vi "Nfocus driver V1.2.vi"(5 "error in":errorcluster, 8 "Refs In":T1) -> (0 "error out":errorcluster)   [LabVIEW 2016]
panel:
  out "Running":bool
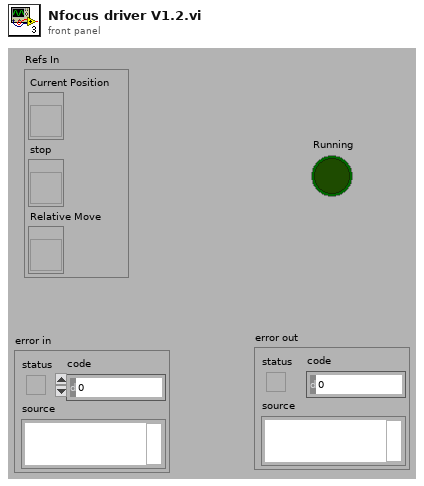
[diagram p1: front panel]
types:
  T1 = cluster{"Current Position":refnum<vi>, "stop":refnum<vi>, "Relative Move":refnum<vi>}
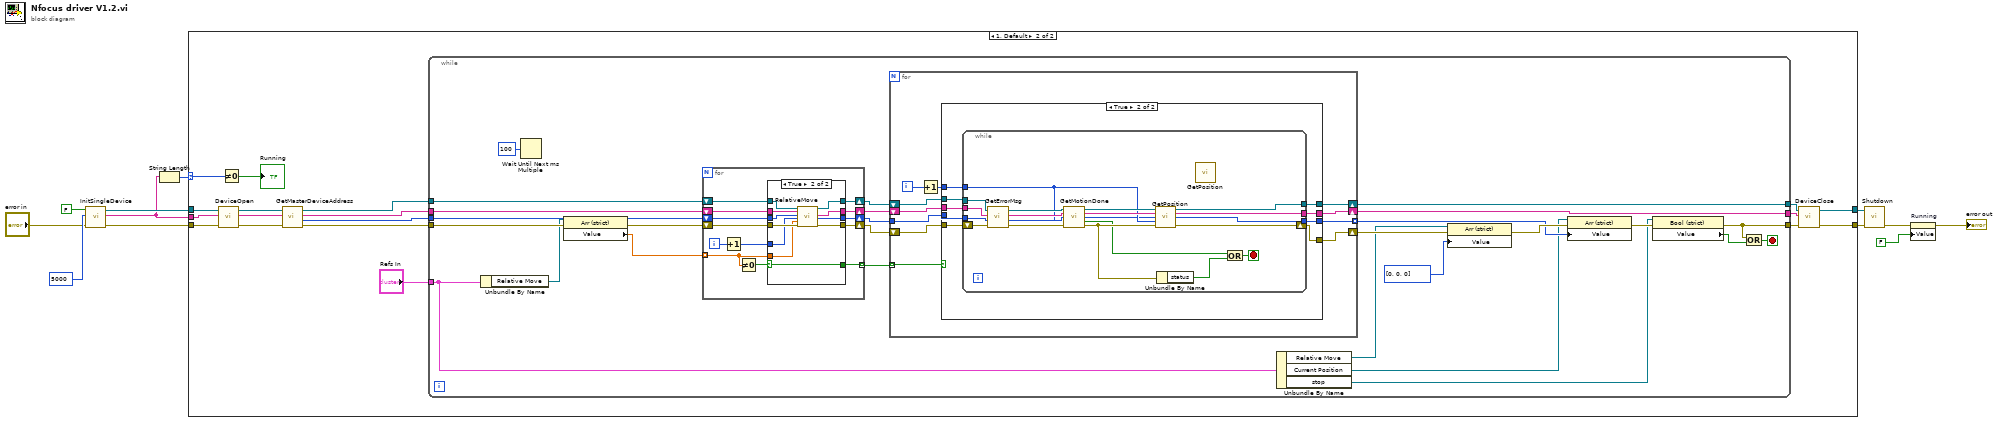
[diagram p0: block diagram]
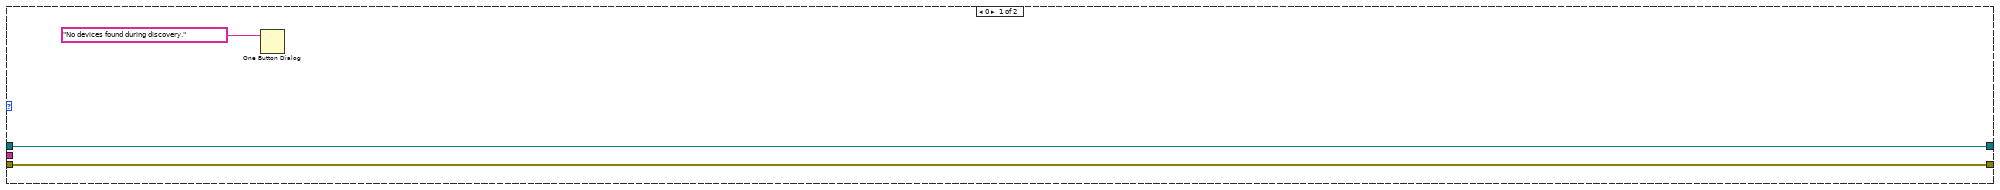
[diagram p2: hidden frame]
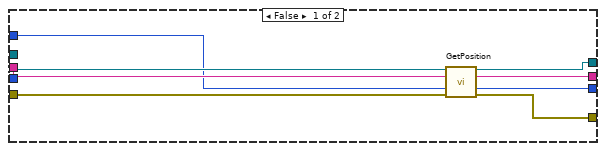
[diagram p4: hidden frame]
diagram:
  n1 = call "InitSingleDevice.vi"("error in (no error)"="error in", "msecDelayForDiscovery"=5000, "logging"=FALSE) -> ("error out"=w5:errorcluster, "DeviceKey Out"=w6:string, "CmdLib Out"=w8:refnum<k24>)  [unwired: 2 in]
  n2 = String Length(string=w6) -> (length=w7:i32)
  n3 = case shown="1, Default" w7 {
    selector: w7 -> [_ w18]
    tunnel: [w14 w20] -> w10
    tunnel: [w13 w22] -> w9
    tunnel: w8 -> [w14 w26]
    tunnel: w6 -> [_ w28]
    tunnel: w5 -> [w13 w30]
    frame 0 {
      n4 = One Button Dialog(message="No devices found during discovery.") -> ()  [unwired: 1 in, 1 out]
    }
    frame 1, Default {
      n5 = call "DeviceOpen.vi"("error in (no error)"=w30, "DeviceKey In"=w28, "CmdLib In"=w26) -> ("error out"=w29:errorcluster, "DeviceKey Out"=w27:string, "CmdLib Out"=w25:refnum<k24>)  [unwired: 2 in]
      n6 = Not Equal To 0?(x=w18) -> (x != 0?=→"Running":bool)
      n7 = call "GetMasterDeviceAddress.vi"("error in (no error)"=w29, "DeviceKey In"=w27, "CmdLib In"=w25) -> ("error out"=w19:errorcluster, "Device Address"=w33:i32, "DeviceKey Out"=w31:string, "CmdLib Out"=w32:refnum<k24>)  [unwired: 1 in]
      n8 = while {
        tunnel: w33 -> [w41]
        tunnel: w32 -> [w43]
        tunnel: [w59] -> w21
        tunnel: w19 -> [w55]
        tunnel: [w57] -> w23
        tunnel: w31 -> [w42]
        tunnel: [w60] -> w24
        tunnel: "Refs In" -> [w48]
        stop <- w58 stop-if-true
        n9 = Unbundle By Name(w48) -> ("Relative Move"=w53:refnum<vi>)
        n10 = Wait Until Next ms Multiple(millisecond multiple=u32 100) -> ()  [unwired: 1 out]
        n11 = property class="Arr (strict)"(reference=w53, error in=w55) -> (error out=w40:errorcluster, "Value"=w35:dbl[])  [unwired: 1 out]
        n12 = for {
          shift-right: [w66] -> w36
          shift-left: w43 -> [w73]
          shift-right: [w67] -> w37
          shift-left: w42 -> [w72]
          shift-right: [w68] -> w38
          shift-left: w41 -> [w71]
          shift-right: [w69] -> w39
          shift-left: w40 -> [w70]
          tunnel: w35 -> [w62] mode=indexing
          tunnel: [w61] -> w34 mode=indexing
          i -> [w65]
          n13 = Increment(x=w65) -> (x+1=w64:i32)
          n14 = Not Equal To 0?(x=w62) -> (x != 0?=w63:bool)
          n15 = case shown="True" w63 {
            selector: w63 -> [w74 w79]
            tunnel: w73 -> [w78 w89]
            tunnel: w72 -> [w77 w88]
            tunnel: w71 -> [w76 w87]
            tunnel: w70 -> [w75 w86]
            tunnel: [w75 w85] -> w69
            tunnel: [w76 w84] -> w68
            tunnel: [w77 w83] -> w67
            tunnel: [w78 w82] -> w66
            tunnel: w62 -> [_ w81]
            tunnel: w64 -> [_ w80]
            tunnel: [w74 w79] -> w61
            frame False {
            }
            frame True {
              n16 = call "RelativeMove.vi"("CmdLib In"=w89, "DeviceKey In"=w88, "Device Address In"=w87, "Motor"=w80, "Relative Steps"=w81, "error in (no error)"=w86) -> ("CmdLib Out"=w82:refnum<k24>, "DeviceKey Out"=w83:string, "Device Address Out"=w84:i32, "error out"=w85:errorcluster)  [unwired: 10 in]
            }
          }
        }
        n17 = for {
          shift-right: [w94] -> w54
          shift-left: w39 -> [w98]
          shift-right: [w99] -> w59
          shift-left: w36 -> [w97]
          shift-right: [w100] -> w60
          shift-left: w37 -> [w96]
          tunnel: w38 -> [w95]
          tunnel: [w93] -> w49 mode=indexing
          tunnel: w34 -> [w90] mode=indexing
          i -> [w91]
          n18 = Increment(x=w91) -> (x+1=w92:i32)
          n19 = case shown="True" w90 {
            tunnel: w95 -> [_ w117]
            tunnel: w97 -> [w108 w116]
            tunnel: w96 -> [w107 w115]
            tunnel: [w104 w114] -> w100
            tunnel: [w103 w113] -> w99
            tunnel: w98 -> [w106 w112]
            tunnel: [w105 w111] -> w94
            tunnel: [w102 w110] -> w93
            tunnel: w92 -> [w101 w109]
            frame False {
              n20 = call "GetPosition.vi"("CmdLib In"=w108, "DeviceKey In"=w107, "Motor"=w101, "error in (no error)"=w106) -> ("CmdLib Out"=w103:refnum<k24>, "DeviceKey Out"=w104:string, "Position"=w102:i32, "error out"=w105:errorcluster)  [unwired: 7 in, 1 out]
            }
            frame True {
              n21 = while {
                tunnel: w109 -> [w119]
                tunnel: w116 -> [w134]
                tunnel: w115 -> [w133]
                tunnel: [w128] -> w113
                tunnel: w117 -> [w127]
                shift-right: [w129] -> w111
                shift-left: w112 -> [w132]
                tunnel: [w121] -> w114
                tunnel: [w122] -> w110
                stop <- w125 stop-if-true
                n22 = call "GetErrorMsg.vi"("error in (no error)"=w132, "Device Address In"=w127, "DeviceKey In"=w133, "CmdLib In"=w134) -> ("error out"=w131:errorcluster, "Device Address Out"=w126:i32, "DeviceKey Out"=w136:string, "CmdLib Out"=w135:refnum<k24>)
                n23 = call "GetMotionDone.vi"("CmdLib In"=w135, "DeviceKey In"=w136, "Device Address In"=w126, "Motor"=w119, "error in (no error)"=w131) -> ("CmdLib Out"=w137:refnum<k24>, "DeviceKey Out"=w120:string, "Device Address Out"=w118:i32, "Is Motion Done"=w124:bool, "error out"=w130:errorcluster)  [unwired: 6 in]
                n24 = call "GetPosition.vi"("CmdLib In"=w137, "DeviceKey In"=w120, "Device Address In"=w118, "Motor"=w119, "error in (no error)"=w130) -> ("CmdLib Out"=w128:refnum<k24>, "DeviceKey Out"=w121:string, "Device Address Out"=w122:i32, "error out"=w129:errorcluster)  [unwired: 6 in, 1 out]
                n25 = Unbundle By Name(w130) -> ("status"=w123:bool)
                n26 = call "GetPosition.vi"() -> ()  [unwired: 11 in, 5 out]
                n27 = Compound Arithmetic op=OR(w124, w123) -> (w125:bool)
              }
            }
          }
        }
        n28 = Unbundle By Name(w48) -> ("Relative Move"=w44:refnum<vi>, "Current Position"=w47:refnum<vi>, "stop"=w46:refnum<vi>)
        n29 = property class="Arr (strict)"(reference=w44, error in=w54, "Value"=i32[] [0, 0, 0]) -> (error out=w51:errorcluster)  [unwired: 1 out]
        n30 = property class="Arr (strict)"(reference=w47, error in=w51, "Value"=w49) -> (error out=w50:errorcluster)  [unwired: 1 out]
        n31 = property on="Property Node" class="Bool (strict)"(reference=w46, error in=w50) -> (error out=w57:errorcluster, "Value"=w56:bool)  [unwired: 1 out]
        n32 = Compound Arithmetic op=OR(w57, w56) -> (w58:bool)
      }
      n33 = call "DeviceClose.vi"("error in (no error)"=w23, "DeviceKey In"=w24, "CmdLib In"=w21) -> ("error out"=w22:errorcluster, "CmdLib Out"=w20:refnum<k24>)  [unwired: 2 in, 1 out]
    }
  }
  n34 = call "Shutdown.vi"("error in (no error)"=w9, "CmdLib In"=w10) -> ("error out"=w3:errorcluster)  [unwired: 4 in, 1 out]
  n35 = property on="Running" class="Bool (strict)"(error in=w3, "Value"=FALSE ("Boolean")) -> (error out=→"error out":errorcluster)  [unwired: 1 in, 1 out]
